vi "UpdateTagMapString.vi"(8 "error in (no error)":errorcluster, 10 "Tag Map":map{string, string}(c390), 11 "Input String":string) -> (0 "error out":errorcluster, 3 "Output String":string)   [LabVIEW 2019, in "LabErrorUX.lvclass"]
uses:
  LabErrorUX.lvclass
  LabErrorUX.lvclass/LabErrorUX.ctl
  <vilib>/SLL Toolkit/SLL String/SLL String.lvlib
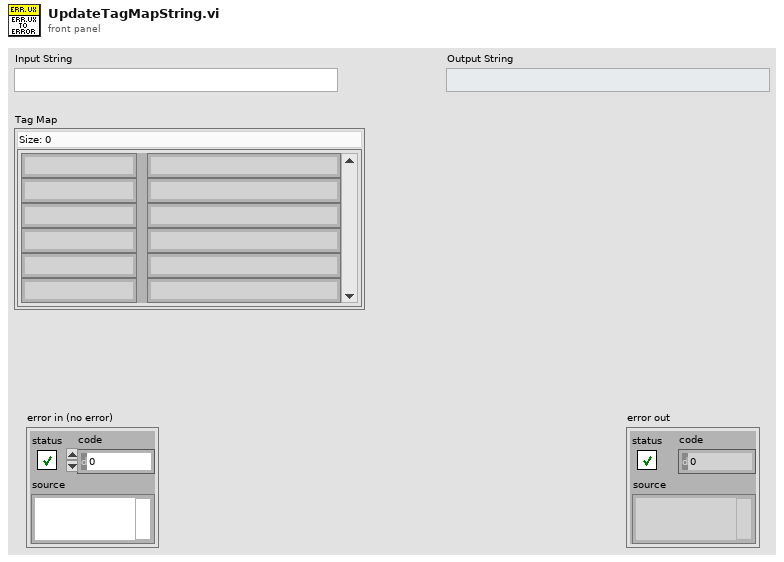
[diagram p1: front panel]
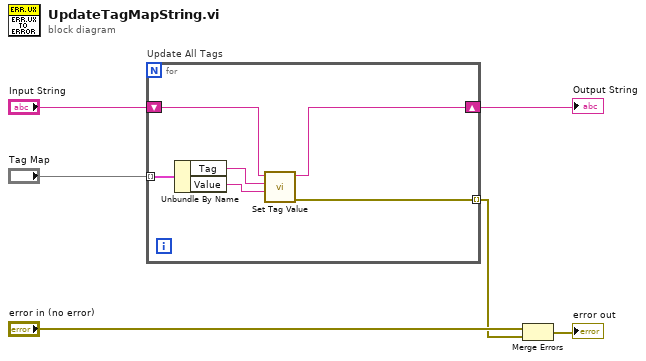
[diagram p0: block diagram]
diagram:
  n1 = for "Update All Tags" {
    tunnel: "Tag Map" -> [w10] mode=indexing
    shift-right: [w11] -> w1
    shift-left: "Input String" -> [w12]
    tunnel: [w7] -> w3 mode=indexing
    n2 = Unbundle By Name(w10) -> ("Tag"=w9:string, "Value"=w8:string)
    n3 = call <vilib>:"Set Tag Value.vi"("Tag Value"=w8, "Tag Name"=w9, "Input String"=w12) -> ("error out"=w7:errorcluster, "Output String"=w11:string)  [unwired: 7 in]
  }
  "Output String" <- w1
  n4 = Merge Errors("error in (no error)", w3) -> (→"error out":errorcluster)
